vi "generateWaveform.vi"(8 "error in (no error)":errorcluster, 11 "TriangleWave in":refnum<class "TriangleWave.lvclass">) -> (0 "error out":errorcluster, 2 "Output":dbl, 3 "TriangleWave out":refnum<class "TriangleWave.lvclass">)   [LabVIEW 2015, in "TriangleWave.lvclass"]
uses:
  TriangleWave.lvclass
  <vilib>/ptbypt/NI_PtbyPt.lvlib
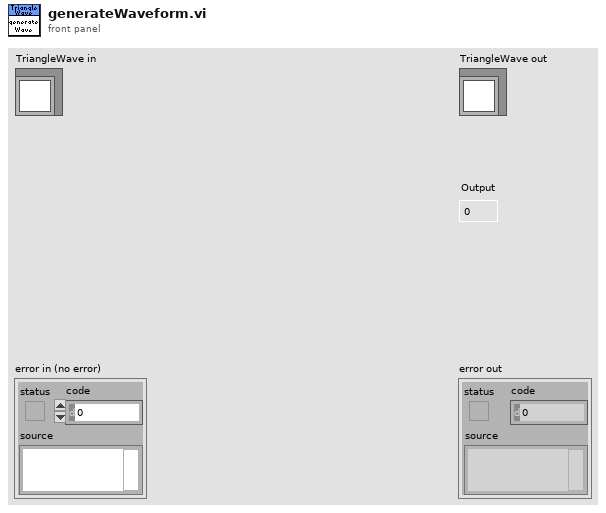
[diagram p1: front panel]
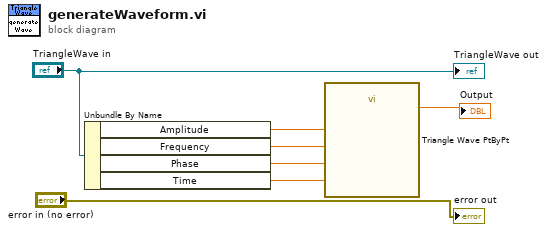
[diagram p0: block diagram]
diagram:
  n1 = Unbundle By Name("TriangleWave in") -> ("Amplitude"=w4:dbl, "Frequency"=w3:dbl, "Phase"=w2:dbl, "Time"=w1:dbl)
  n2 = call <vilib>:"Triangle Wave PtByPt.vi"("time"=w1, "phase"=w2, "frequency"=w3, "amplitude"=w4) -> ("triangle wave"=→"Output":dbl)
  "error out" <- "error in (no error)"
  "TriangleWave out" <- "TriangleWave in"
